vi "Wrapper.vi"(0 "Update Device Setpoint in":refnum<class "Update Device Setpoint.lvclass">, 1 "Actor in":refnum<class "Actor.lvclass">, 5 "error in (no error)":errorcluster) -> (14 "Controller out":refnum<class "Controller.lvclass">, 19 "error out":errorcluster)   [LabVIEW 2014, in "Controller.lvlib" / "Update Device Setpoint.lvclass"]
uses:
  Update Device Setpoint.lvclass
  Controller.lvclass
  <vilib>/ActorFramework/Actor/Actor.lvclass
  Devices/Configurable Device/Actor/Send New Setpoint MSG/Send New Setpoint.lvclass
  Controls/eMap.ctl
  <vilib>/ActorFramework/Message Enqueuer/Message Enqueuer.lvclass
  Controller.lvclass/Controller.ctl
  Update Device Setpoint.lvclass/Update Device Setpoint.ctl
  Devices/Configurable Device/Actor/Send New Setpoint MSG/Send New Setpoint.lvclass/Send New Setpoint.ctl
  <vilib>/ActorFramework/Message Enqueuer/Message Enqueuer.lvclass/Message Enqueuer.ctl
  Devices/Configurable Device/Actor/Send New Setpoint MSG/Write Setpoint.vi
  Accessors/Read Enqueuer Map.vi
  Accessors/Read log.vi
  <vilib>/ActorFramework/Message Priority Queue/Priority Enqueue.vi
  <userlib>/_Session Fwk/Session - Root.lvclass
  reusable/Session APIs/Session Log/System Log.lvclass
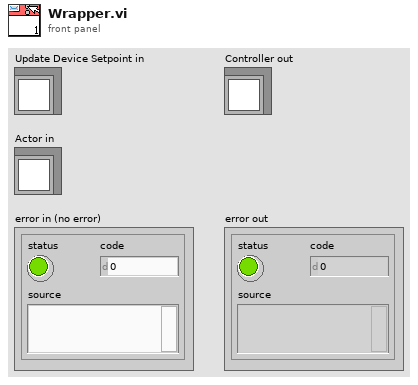
[diagram p1: front panel]
types:
  T1 = typedef "Controller.lvlib/Controller.lvclass/eMap.ctl" = cluster{"Enqueuer":refnum<class "Message Enqueuer.lvclass">, "Active":bool}
  T2 = typedef "Session - Root.lvclass/Session Handle.ctl" = refnum<data-value>
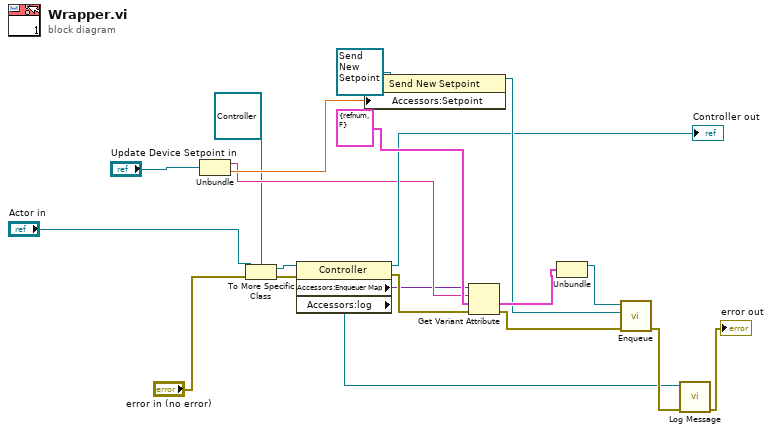
[diagram p0: block diagram]
diagram:
  n1 = Unbundle("Update Device Setpoint in") -> (w11:string, w15:dbl)
  n2 = To More Specific Class(target class=refnum<class "Controller.lvclass"> refnum ("Controller.lvlib:Controller"), reference="Actor in", error in="error in (no error)") -> (specific class reference=w7:refnum<class "Controller.lvclass">, error out=w9:errorcluster)
  n3 = property class="Controller"(reference=w7, error in=w9) -> (reference out=→"Controller out":refnum<class "Controller.lvclass">, error out=w12:errorcluster, "Accessors:Enqueuer Map"=w10:variant, "Accessors:log"=w1:T2)
  n4 = property class="Send New Setpoint"(reference=refnum<class "Send New Setpoint.lvclass"> refnum ("Device.lvlib:Send New Setpoint"), "Accessors:Setpoint"=w15) -> (reference out=w16:refnum<class "Send New Setpoint.lvclass">)  [unwired: 1 in, 1 out]
  n5 = Get Variant Attribute(Variant=w10, name=w11, default value (empty Variant)=T1 {"Enqueuer"=refnum, "Active"=FALSE} ("eMap"), error in=w12) -> (value=w19:T1, error out=w17:errorcluster)  [unwired: 2 out]
  n6 = Unbundle(w19) -> ("Enqueuer"=w20:refnum<class "Message Enqueuer.lvclass">)  [unwired: 1 out]
  n7 = call <vilib>:"Enqueue.vi"("error in (no error)"=w17, "Message"=w16, "Message Enqueuer in"=w20) -> ("error out"=w3:errorcluster)  [unwired: 7 in, 1 out]
  n8 = call "Log Message.vi"("error in"=w3, "session in"=w1) -> ("error out"=→"error out":errorcluster)  [unwired: 8 in, 1 out]
